vi "mes~KPSN_Input.vi"(8 "错误输入（无错误）":errorcluster, 10 "sn":string, 11 "wo":string) -> (0 "错误输出":errorcluster, 1 "Message":string, 2 "KPSN_OK":bool)   [LabVIEW 2015]
uses:
  ctl/KPSN_Input.ctl
  Global.vi
panel:
  in  "Headers":string[][](array[string])=[["Content-Type", "text/xml;charset=UTF-8"], ["SOAPAction", "\"MesWebService/KPSN_Input\""], ["Host", "10.32.12.103"]]
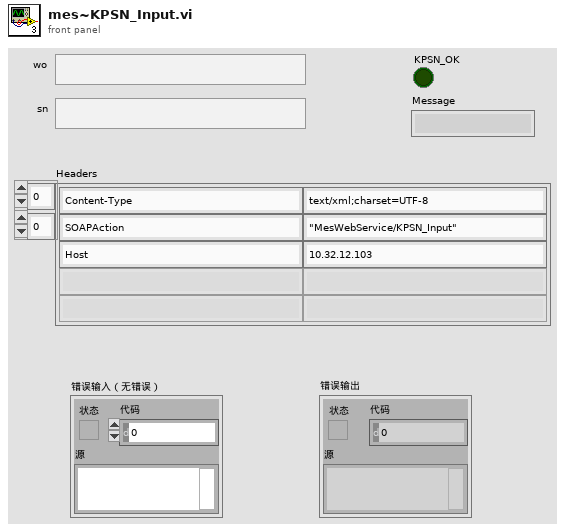
[diagram p1: front panel]
types:
  T1 = typedef "KPSN_Input.ctl" = cluster{"#attributes":cluster{"xmlns:xsi":string, "xmlns:xsd":string, "xmlns:soap":string}, "soap:Body":cluster{"KPSN_Input":cluster{"#attributes":cluster{"xmlns":string}, "sn":string, "wo":string}}}
  T2 = cluster{"URL":string, "audit_mode":string, "tsid":string, "model":string, "product":string, "test_station":string, "station_id":string, "test_station_name":string, "Webservice":string}
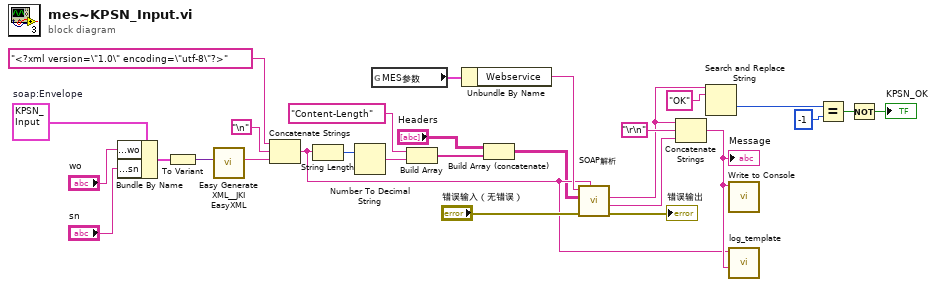
[diagram p0: block diagram]
diagram:
  w9 = T1 {"#attributes"={"xmlns:xsi"="http://www.w3.org/2001/XMLSchema-instance", "xmlns:xsd"="http://www.w3.org/2001/XMLSchema", "xmlns:soap"="http://schemas.xmlsoap.org/soap/envelope/"}, "soap:Body"={"KPSN_Input"={"#attributes"={"xmlns"="MeswebService"}, "sn"="", "wo"=""}}}  # soap:Envelope
  n1 = Bundle By Name(cluster=w9, "soap:Body.KPSN_Input.wo"="wo", "soap:Body.KPSN_Input.sn"="sn") -> (w28:T1)
  n2 = To Variant(anything=w28) -> (Variant=w27:variant)
  n3 = call <vilib>:"Easy Generate XML__JKI EasyXML.vi"("LabVIEW Data"=w27) -> ("XML String"=w12:string)  [unwired: 9 in, 1 out]
  n4 = Concatenate Strings("<?xml version=\"1.0\" encoding=\"utf-8\"?>" ("字符串"), "\n", w12) -> (w7:string)
  n5 = String Length(string=w7) -> (length=w6:i32)
  n6 = Number To Decimal String(number=w6) -> (decimal integer string=w5:string)  [unwired: 1 in]
  n7 = global read "Global.vi" "MES参数"() -> (w4:T2)
  n8 = Build Array("Content-Length" ("字符串"), w5) -> (w2:string[])
  n9 = Unbundle By Name(w4) -> ("Webservice"=w24:string)
  n10 = Build Array (concatenate)("Headers", w2) -> (w1:string[][])
  n11 = call "SOAP解析.vi"("DATA"=w7, "错误输入（无错误）"="错误输入（无错误）", "Headers"=w1, "URL"=w24) -> ("错误输出"=→"错误输出":errorcluster, "body"=w22:string, "headers"=w21:string)  [unwired: 5 in]
  n12 = Concatenate Strings(w21, "\r\n", w22) -> (w13:string)
  "Message" <- w13
  n13 = Search and Replace String(input string=w21, search string="OK" ("搜索字符串")) -> (offset past replacement=w19:i32)  [unwired: 6 in, 3 out]
  n14 = call "Write to Console.vi"("Input"=w13) -> ()  [unwired: 10 in, 1 out]
  n15 = call "log_template.vi"("接收报文"=w13, "发送报文"=w7) -> ()  [unwired: 10 in]
  n16 = Equal?(x=w19, y=-1) -> (x = y?=w17:bool)
  n17 = Not(x=w17) -> (.not. x?=→"KPSN_OK":bool)
